vi "Volt to Distance.vi"(1 "Calibration Parameters":T1, 2 "Voltage":fxp<+/-,26,5>) -> (0 "Distance":fxp<+/-,26,5>)   [LabVIEW 2012]
panel:
  # "Convert Sharp IR voltage to range"
types:
  T1 = cluster{"m":fxp<+/-,26,5>, "b":fxp<+/-,26,5>, "k":fxp<+/-,26,5>}
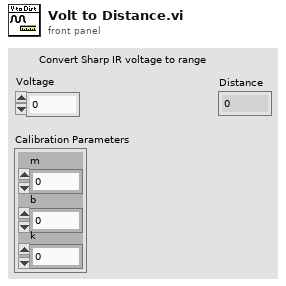
[diagram p1: front panel]
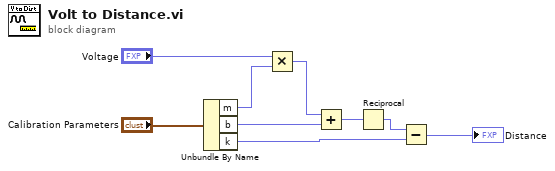
[diagram p0: block diagram]
diagram:
  n1 = Unbundle By Name("Calibration Parameters") -> ("m"=w8:fxp<+/-,26,5>, "b"=w6:fxp<+/-,26,5>, "k"=w7:fxp<+/-,26,5>)
  n2 = Multiply(x="Voltage", y=w8) -> (x*y=w5:fxp<+/-,52,10>)
  n3 = Add(x=w5, y=w6) -> (x+y=w3:fxp<+/-,26,5>)
  n4 = Reciprocal(x=w3) -> (1/x=w4:fxp<+/-,26,5>)
  n5 = Subtract(x=w4, y=w7) -> (x-y=→"Distance":fxp<+/-,26,5>)
